vi "dome_cancelCallback_command_enableackcmd.vi"(8 "error in (no error)":errorcluster) -> (0 "error out":errorcluster, 3 "function return":i32)   [LabVIEW 2016, in "SALLV_dome.lvlib"]
doc: "int dome_shm_cancelCallback_command_enable_ackcmdLV();"
uses:
  SALLV_dome.lvlib
  SALLV_dome.so
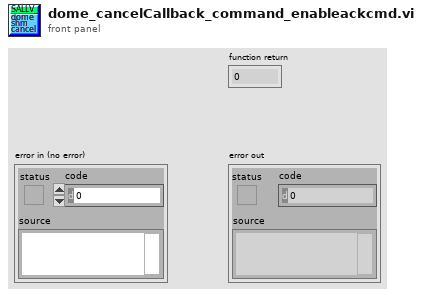
[diagram p1: front panel]
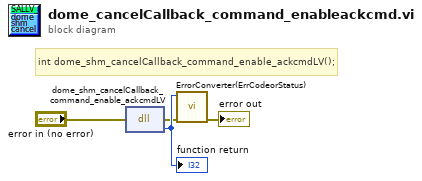
[diagram p0: block diagram]
diagram:
  # "int dome_shm_cancelCallback_command_enable_ackcmdLV();"
  n1 = dll-call lib="home/andres/Desktop/SALLV_dome/SALLV_dome.*" fn="dome_shm_cancelCallback_command_enable_ackcmdLV"(error in="error in (no error)") -> (error out=w2:errorcluster, w4:i32)  [unwired: 2 in, 1 out]
  "function return" <- w4
  n2 = call "ErrorConverter(ErrCodeorStatus).vi"("error in (no error)"=w2, "error code"=w4) -> ("error out"=→"error out":errorcluster)  [unwired: 9 in]
